vi "sendSignal.vi"(8 "error in (no error)":errorcluster, 11 "Dectrum12A in":refnum<class "Dectrum12A.lvclass">) -> (0 "error out":errorcluster, 3 "Dectrum12A out":refnum<class "Dectrum12A.lvclass">)   [LabVIEW 2015, in "Dectrum12A.lvclass"]
uses:
  Dectrum12A.lvclass
  Dectrum12A.lvclass/Dectrum12A.ctl
panel:
  in  "Throttle [%]":dbl
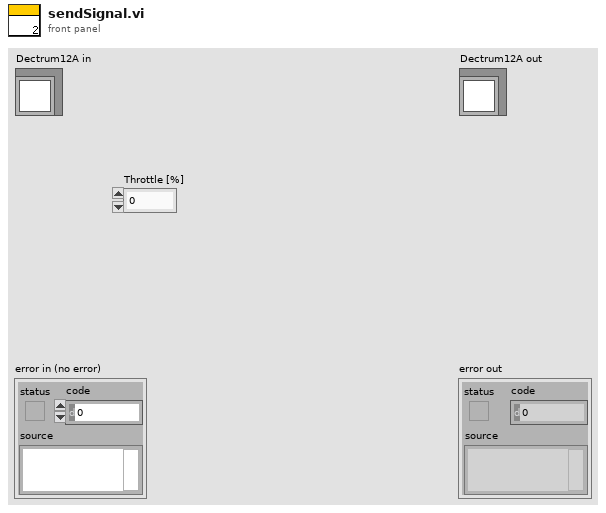
[diagram p1: front panel]
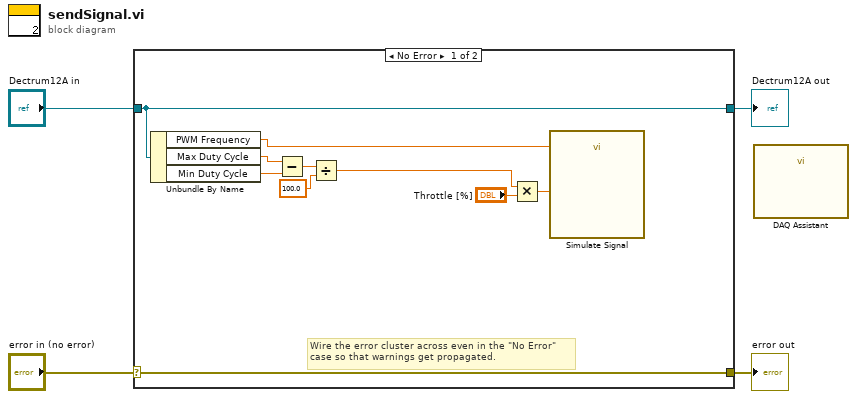
[diagram p0: block diagram]
diagram:
  n1 = case shown="No Error" "error in (no error)" {
    selector: "error in (no error)" -> [w14 w16]
    tunnel: [w14 w16] -> w3
    tunnel: [w13 w15] -> w1
    tunnel: "Dectrum12A in" -> [w13 w15]
    frame No Error {
      # "Wire the error cluster across even in the \"No Error\"\ncase so that warnings get propagated."
      n2 = Unbundle By Name(w13) -> ("PWM Frequency"=w5:dbl, "Max Duty Cycle"=w7:dbl, "Min Duty Cycle"=w6:dbl)
      n3 = Subtract(x=w7, y=w6) -> (x-y=w12:dbl)
      n4 = Divide(x=w12, y=100.0) -> (x/y=w8:dbl)
      n5 = Multiply(x=w8, y="Throttle [%]") -> (x*y=w10:dbl)
      n6 = call "Simulate Signal"("Duty Cycle (%)"=w10, "Frequency"=w5) -> ()  [unwired: 12 in, 2 out]
    }
    frame Error {
    }
  }
  "error out" <- w3
  "Dectrum12A out" <- w1
  n7 = call "DAQ Assistant"() -> ()  [unwired: 17 in, 3 out]
